vi "Test Normal Coefficient of Variation PDF.vi"() -> ()   [LabVIEW 2021, in "Math.lvlib"]
uses:
  Fits/Fit Settings.ctl
  Fits/Nonlinear Fit Method.ctl
  Fits/Ramp Type.ctl
  Fits/Residual Type.ctl
  Fits/Non-linear Fitting Algorithm.ctl
  Fits/Fit Plot Request Information.ctl
  <vilib>/Utility/miscctls.llb/LVPointDoubleTypeDef.ctl
  Fits/Fit Models.ctl
  85f3da7c-8858-4d9f-a12c-d9901bcd4fde.vi
  Math.lvlib
  Fits/Fits.lvlib
panel:
  out "error out":errorcluster={"status"=FALSE, "code"=-23026, "source"="Scale range exceeded"}
  in  "Fit Settings":T1={"Use Original Plot # Points"=TRUE, "# Fit Plot Points"=0, "Fitting Method"=enum."Least Square", "Weighted Fit"=FALSE, "Show All Fit Components"=FALSE, "Axis Type"=0, "Show Fit Residuals"=TRUE, "Residual Type"=enum."Standard", "Fitting Algorithm"=enum."Levenberg-Marquardt"} {"Axis Type" items=["Linear", "Logarithmic"]}
  out "Fit Result String":string="CV PDF  Gaussian LM Least Square Fit:\nAmplitude: 25.528592 ± 0.013986\nCenter: 0.210423 ± 9.838581E-6\nSDV: 0.015489 ± 9.825245E-6\nFWHM: 0.036473 ± 2.313668E-5\nIntegral: 991.140471\nMSE: 0.060195\nR^2: 0.999786\n"
  out "XY Graph":cluster{"X Array":dbl[], "Y Array":dbl[]}[](graph)
  in  "n":i32=100
  in  "CV":dbl=0.21
  in  "# Steps (1)":i32=1000
  in  "End (1)":dbl=1.0
  in  "Start (0)":dbl
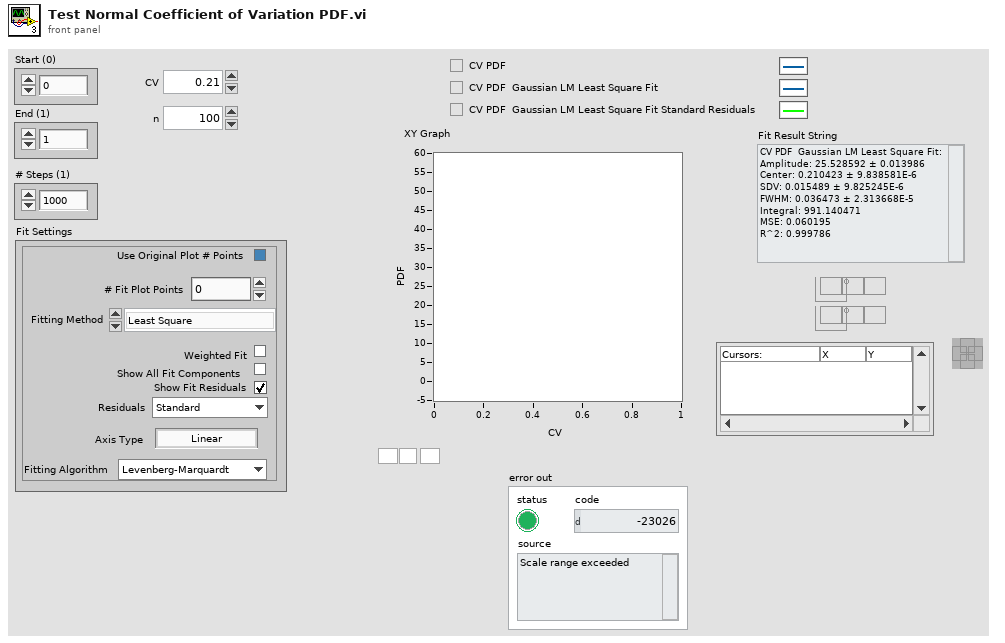
[diagram p1: front panel]
types:
  T1 = typedef "Fits.lvlib/Fit Settings.ctl" = cluster{"Use Original Plot # Points":bool, "# Fit Plot Points":u32, "Fitting Method":T2, "Weighted Fit":bool, "Show All Fit Components":bool, "Axis Type":T3, "Show Fit Residuals":bool, "Residual Type":T4, "Fitting Algorithm":T5}
  T2 = typedef "Fits.lvlib/Nonlinear Fit Method.ctl" = enum16{"Least Square", "Least Absolute Residual", "Bisquare", "MLE"}
  T3 = typedef "Fits.lvlib/Ramp Type.ctl" = u16
  T4 = typedef "Fits.lvlib/Residual Type.ctl" = enum16{"Standard", "Normalized", "Reduced"}
  T5 = typedef "Fits.lvlib/Non-linear Fitting Algorithm.ctl" = enum16{"Levenberg-Marquardt", "Trust-Region Dogleg"}
  T6 = typedef "LVPointDoubleTypeDef.ctl" = cluster{"X":dbl, "Y":dbl}
  T7 = typedef "Fits.lvlib/Fit Models.ctl" = enum16{"Select a Fit Model...", "           Single Peak", "Gaussian", "Asymmetric Gaussian", "Lorentzian", "Asymmetric Lorentzian", "Gaussian/Lorentzian", "Lorentzian/Gaussian", "           Double Peak", "Two Gaussians", "Two Asymmetric Gaussians", "Two H-Connected Gaussians", "Two T-Connected Gaussians", "Two H-Connected Asymmetric Gaussians", "Two T-Connected Asymmetric Gaussians", "           Triple Peak", "Three Gaussians", "Three Asymmetric Gaussians", "              Decays", "1-Exponential", "IRF*PSED", "2-Exponentials", "            Power Law", "Power Law", "Power Law with Offset", "Power Law from Intensity Distribution", "               ACF", "2D Gaussian ACF", "2D Gaussian + Blinking ACF", "2D Gaussian + Flow ACF", "3D Gaussian ACF", "3D Gaussian + Blinking ACF", "             Multiplot", "2D Gaussian ACF & 2D Gaussian + Flow ACF"}
  T8 = typedef "Fits.lvlib/Fit Plot Request Information.ctl" = cluster{"XY Graph Ref":refnum<vi>, "Mouse Coordinates":T6, "Fit Model":T7, "Plot Index":i32}
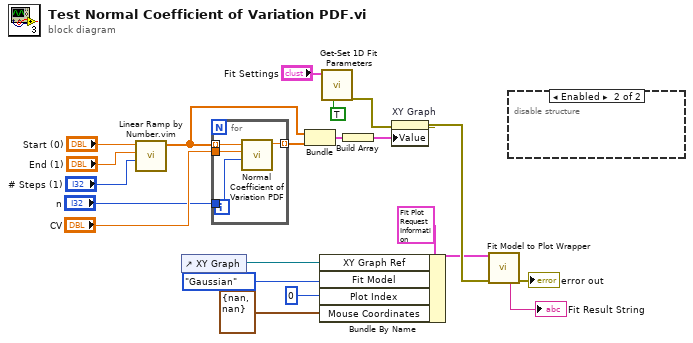
[diagram p0: block diagram]
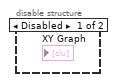
[diagram p2: hidden frame]
diagram:
  n1 = call "Linear Ramp by Number.vim"("# Steps (1)"="# Steps (1)", "End (1)"="End (1)", "Start (0)"="Start (0)") -> ("Ramp"=w15:dbl[])  [unwired: 6 in, 2 out]
  n2 = control-ref of="XY Graph"() -> (w9:refnum<vi>)
  n3 = for {
    tunnel: w15 -> [w25] mode=indexing
    tunnel: "CV" -> [w24]
    tunnel: "n" -> [w23]
    tunnel: [w22] -> w16 mode=indexing
    n4 = call "Normal Coefficient of Variation PDF.vi"("n"=w23, "CV"=w24, "x"=w25) -> ("PDF (x)"=w22:dbl)  [unwired: 7 in, 1 out]
  }
  n5 = Bundle("Ramp"=w15, w16) -> (w14:cluster{"Ramp":dbl[], dbl[]})  [unwired: 1 in]
  n6 = Bundle By Name(cluster=T8 {"XY Graph Ref"=refnum, "Mouse Coordinates"={"X"=0.0, "Y"=0.0}, "Fit Model"=enum."Gaussian", "Plot Index"=0} ("Fit Plot Info"), "XY Graph Ref"=w9, "Fit Model"=Fit_Models."Gaussian", "Plot Index"=0, "Mouse Coordinates"=T6 {"X"=nan, "Y"=nan}) -> (w10:T8)
  n7 = call "Get-Set 1D Fit Parameters.vi"("Get(F)/Set"=TRUE, "Fit Settings"="Fit Settings") -> ("Error Out"=w1:errorcluster)  [unwired: 6 in, 3 out]
  n8 = Build Array(w14) -> (w12:cluster{"Ramp":dbl[], dbl[]}[])
  n9 = property on="XY Graph" class="XYGraph (strict)"(error in=w1, "Value"=w12) -> (error out=w11:errorcluster)  [unwired: 1 in, 1 out]
  n10 = call "Fit Model to Plot Wrapper.vi"("Fit Plot Info"=w10, "error in (no error)"=w11) -> ("Fit Result String"=→"Fit Result String":string, "error out"=→"error out":errorcluster)  [unwired: 5 in, 7 out]
  n11 = disable-structure shown="Enabled" {
    frame Disabled {
    }
    frame Enabled {
    }
  }
